vi "GPIB Command.vi"(0 "GPIB (In)":cluster{"GPIB address":i16, "GPIB bus":i16}={"GPIB address"=22, "GPIB bus"=0}, 1 "Input command":string, 2 "error in":T1) -> (3 "GPIB (Out)":cluster{"GPIB address":i16, "GPIB bus":i16}={"GPIB address"=22, "GPIB bus"=0}, 4 "Bytes sent":i32, 5 "Return string":string, 6 "error out":T1)   [LabVIEW 2018]
doc: "Implements a GPIB command given the GPIB bus information and the input command string. The *OPC? query is sent after each command for handshaking purposes.\n\nMultiple serial polls are performed as required after sending the *OPC? command in order to determine when bit 4 (GPIB MESSAGE AVAILABLE) is set indicating the return data is available. Instruments must support the IEEE 488.2 spec for the serial poll byte for this VI to work correctly.\n\nThe *OPC? timeout setting (internal to VI) limits the amount of time the VI will wait for bit 4 to be set by the instrument."
panel:
  in  "*OPC? timeout (sec)":dbl=2.0 format="%.2f"
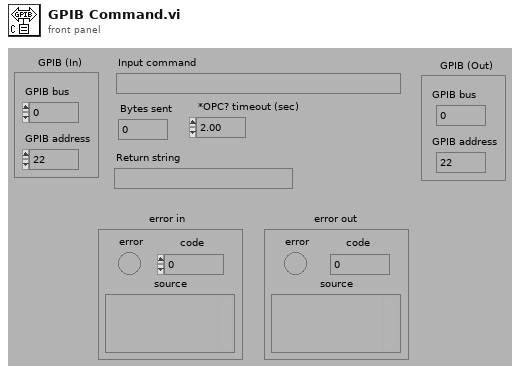
[diagram p1: front panel]
types:
  T1 = cluster{"error":bool, "code":i32, "source":string}
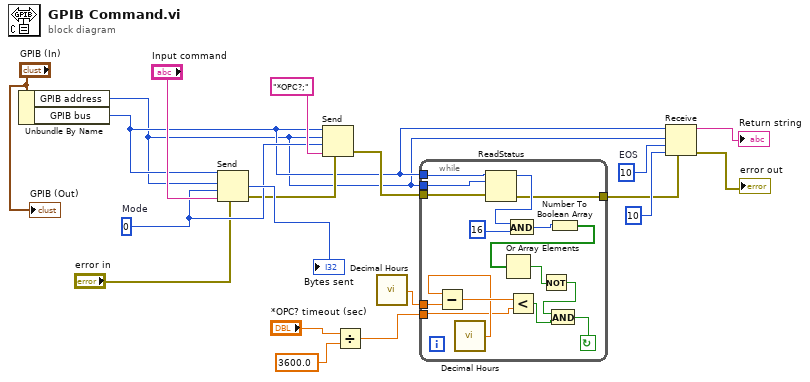
[diagram p0: block diagram]
diagram:
  w1 = u8 10  # EOS
  w11 = u8 0  # Mode
  n1 = Unbundle By Name("GPIB (In)") -> ("GPIB address"=w3:i16, "GPIB bus"=w4:i16)
  n2 = Send(0:w4, 2:w3, 3:w11, 4:"error in", 5:"Input command") -> (7:→"Bytes sent":i32, 8:w9:errorcluster)  [unwired: 1 out]
  n3 = Send(0:w4, 2:w3, 3:w11, 4:w9, 5:"*OPC?;") -> (8:w7:errorcluster)  [unwired: 2 out]
  n4 = Divide(x="*OPC? timeout (sec)", y=3600.0) -> (x/y=w8:dbl)
  n5 = call "Decimal Hours.vi"() -> ("decimal hours now"=w13:dbl)  [unwired: 2 in]
  n6 = while {
    tunnel: [w20] -> w2
    tunnel: w7 -> [w21]
    tunnel: w13 -> [w22]
    tunnel: w8 -> [w23]
    tunnel: w4 -> [w34]
    tunnel: w3 -> [w35]
    stop <- w24 continue-if-true
    n7 = call "Decimal Hours.vi"() -> ("decimal hours now"=w27:dbl)  [unwired: 2 in]
    n8 = Subtract(x=w27, y=w22) -> (x-y=w28:dbl)
    n9 = ReadStatus(3:w21, 4:w35, 5:w34) -> (0:w20:errorcluster, 2:w33:i16)  [unwired: 1 out]
    n10 = And(x=w33, y=i16 16) -> (x .and. y?=w31:i16)
    n11 = Less?(x=w28, y=w23) -> (x < y?=w26:bool)
    n12 = Number To Boolean Array(number=w31) -> (Boolean array=w30:bool[])
    n13 = Or Array Elements(Boolean array=w30) -> (logical OR=w29:bool)
    n14 = Not(x=w29) -> (.not. x?=w25:bool)
    n15 = And(x=w25, y=w26) -> (x .and. y?=w24:bool)
  }
  n16 = Receive(4:w2, 6:10, 7:w1, 8:w3, 9:w4) -> (0:→"error out":errorcluster, 3:→"Return string":string)  [unwired: 2 out]
  "GPIB (Out)" <- "GPIB (In)"
